vi "InstanceDestroy.vi"(8 "error in (no error)":errorcluster, 11 "Singleton.lvclass In":refnum<class "Singleton.lvclass">) -> (0 "error out":errorcluster, 3 "Singleton.lvclass Out":refnum<class "Singleton.lvclass">)   [LabVIEW 2014, in "Singleton.lvclass"]
uses:
  Singleton.lvclass
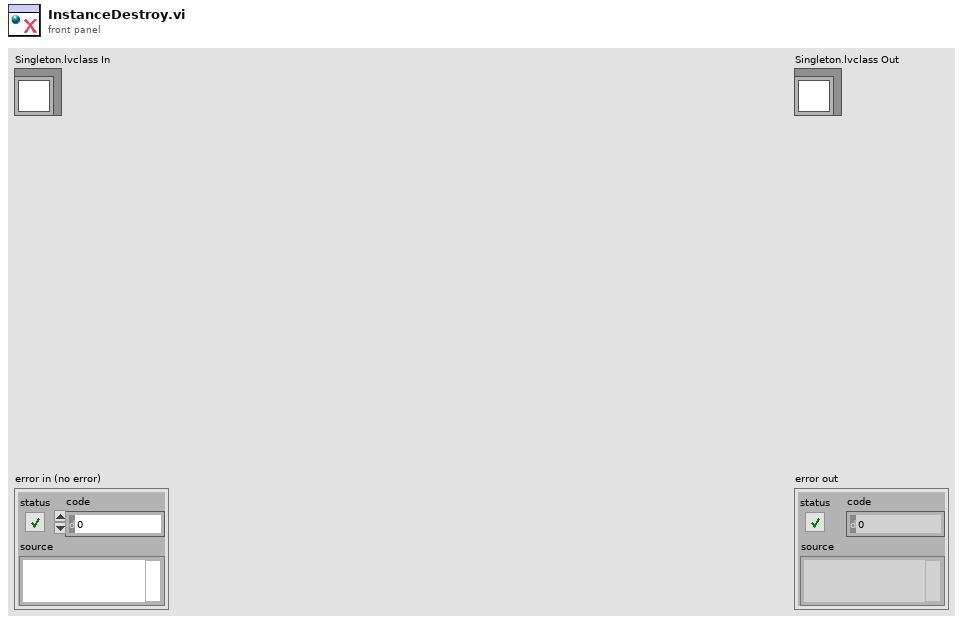
[diagram p1: front panel]
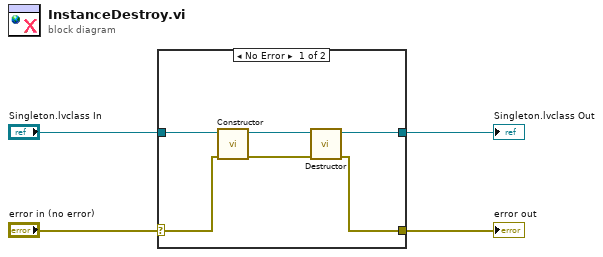
[diagram p0: block diagram]
diagram:
  n1 = case shown="No Error" "error in (no error)" {
    selector: "error in (no error)" -> [w8 w12]
    tunnel: [w7 w12] -> w3
    tunnel: [w6 w11] -> w1
    tunnel: "Singleton.lvclass In" -> [w5 w11]
    frame No Error {
      n2 = call "Constructor.vi"("error in (no error)"=w8, "Singleton.lvclass In"=w5) -> ("error out"=w10:errorcluster, "SingletonDVR Out"=w9:refnum<data-value>)  [unwired: 8 in]
      n3 = call "Destructor.vi"("error in (no error)"=w10, "SingletonDVR In"=w9) -> ("error out"=w7:errorcluster, "Singleton.lvclass Out"=w6:refnum<class "Singleton.lvclass">)  [unwired: 8 in]
    }
    frame Error {
    }
  }
  "error out" <- w3
  "Singleton.lvclass Out" <- w1
